vi "Trigger Force.vi"   [LabVIEW 2021, in "vmmso.lvlib"]
doc: "DLL_API void WINAPI TriggerForce();"
uses:
  vmmso.lvlib
  vmmso.dll
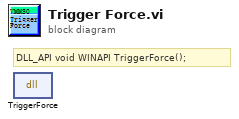
[diagram p0: block diagram]
diagram:
  # "DLL_API void WINAPI TriggerForce();"
  n1 = dll-call lib="D:/labviewdemo/LabviewDemo 21/vmmso/vmmso.*" fn="TriggerForce"() -> ()  [unwired: 4 in, 2 out]
